vi "GetNetworkData.vi"(0 "TCP Network Connection in":refnum<k5>, 11 "error in (no error)":errorcluster) -> (4 "TCP Network Connection out":refnum<k5>, 6 "console":string, 8 "sensors":dbl[](array[numeric]), 10 "states":i32[](array[numeric]), 15 "error out":errorcluster)   [LabVIEW 2022 SP3]
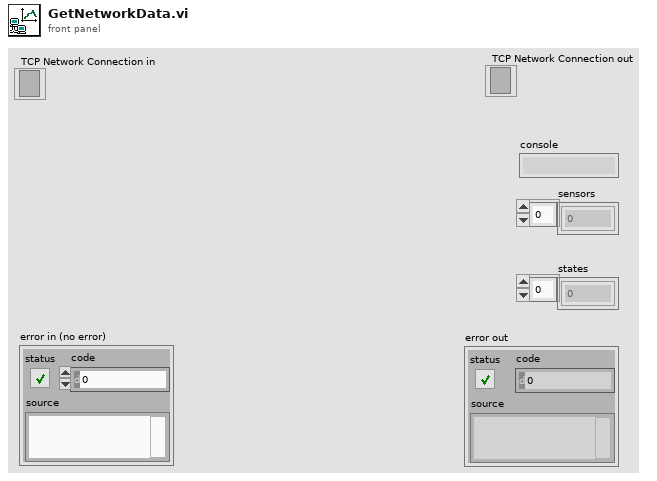
[diagram p1: front panel]
types:
  T1 = cluster{"states":i32[], "timestamp":string, "console":string, "sensors":dbl[]}
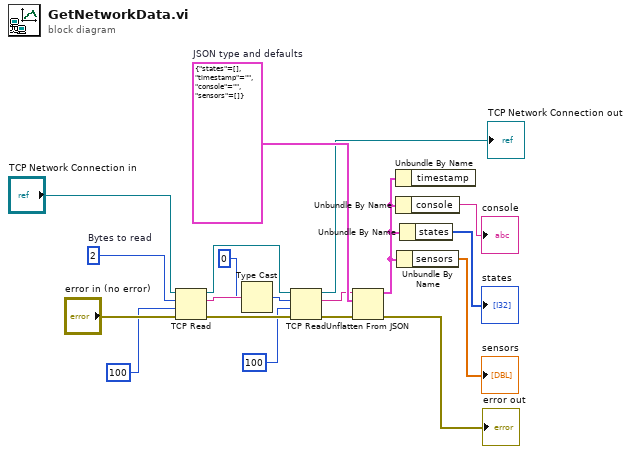
[diagram p0: block diagram]
diagram:
  w13 = T1 {"states"=[], "timestamp"="", "console"="", "sensors"=[]}  # JSON type and defaults
  w5 = 2  # Bytes to read
  n1 = TCP Read(connection ID="TCP Network Connection in", bytes to read=w5, error in (no error)="error in (no error)", 9:100) -> (connection ID out=w18:refnum<k5>, data out=w8:string, error out=w6:errorcluster)  [unwired: 1 in]
  n2 = Type Cast(type=u16 0, x=w8) -> (*(type *) &x=w19:u16)
  n3 = TCP Read(connection ID=w18, bytes to read=w19, error in (no error)=w6, 9:100) -> (connection ID out=→"TCP Network Connection out":refnum<k5>, data out=w10:string, error out=w11:errorcluster)  [unwired: 1 in]
  n4 = Unflatten From JSON(JSON string=w10, type and defaults=w13, error in (no error)=w11) -> (value=w9:T1, error out=→"error out":errorcluster)  [unwired: 4 in]
  n5 = Unbundle By Name(w9) -> ()  [unwired: 1 out]
  n6 = Unbundle By Name(w9) -> ("console"=→"console":string)
  n7 = Unbundle By Name(w9) -> ("sensors"=→"sensors":dbl[])
  n8 = Unbundle By Name(w9) -> ("states"=→"states":i32[])
